vi "Get Channel Group.vi"   [LabVIEW 2026, in "Template Plugin.lvlib" / "Template.lvclass"]
uses:
  Template.lvclass
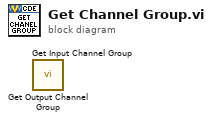
[diagram p0: block diagram]
diagram:
  n1 = call "Get Output Channel Group.vi"() -> ()  [unwired: 9 in, 3 out]
  n2 = call "Get Input Channel Group.vi"() -> ()  [unwired: 9 in, 3 out]
